vi "MeasurementSpin2String.vi"(1 "Seconds after Spin Stop":dbl[unit]=1.0, 2 "Seconds to Spin Start":dbl[unit]=1.0, 3 "Program Spin Coater":T1(array[cluster])) -> (0 "concatenated string":string)   [LabVIEW 2020]
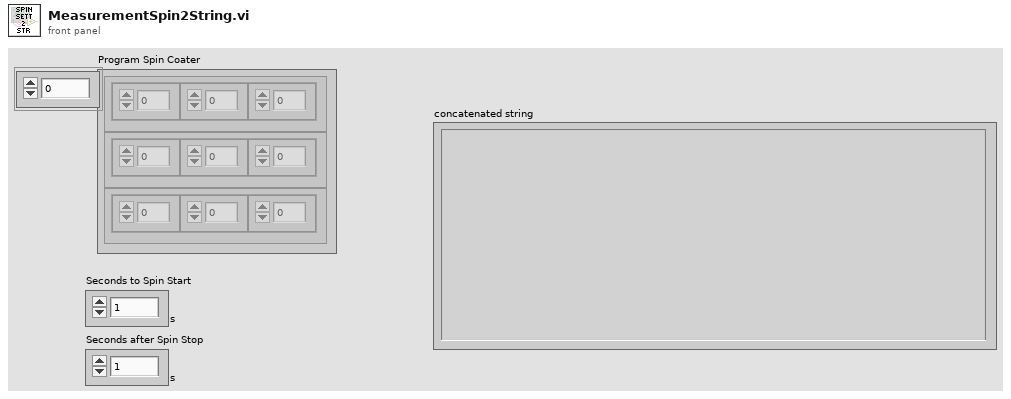
[diagram p1: front panel]
types:
  T1 = cluster{"Speed (rpm)":dbl, "Time (s)":dbl, "Acc (rpm/s)":dbl}[]
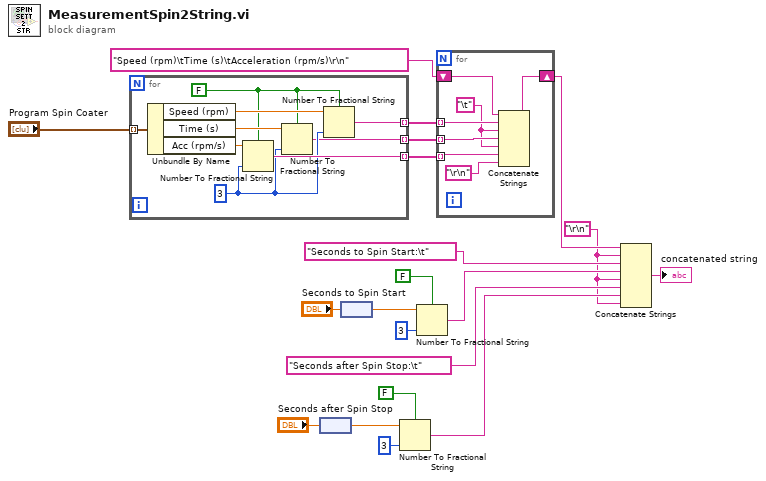
[diagram p0: block diagram]
diagram:
  w2 = "\r\n"
  n1 = for {
    tunnel: [w29] -> w19 mode=indexing
    tunnel: [w28] -> w17 mode=indexing
    tunnel: "Program Spin Coater" -> [w26] mode=indexing
    tunnel: [w23] -> w18 mode=indexing
    w27 = i16 3 ("precision (6)")
    w21 = FALSE ("use system decimal point (T)")
    n2 = Unbundle By Name(w26) -> ("Speed (rpm)"=w25:dbl, "Time (s)"=w24:dbl, "Acc (rpm/s)"=w22:dbl)
    n3 = Number To Fractional String(use system decimal point (T)=w21, number=w22, precision (6)=w27) -> (F-format string=w28:string)  [unwired: 1 in]
    n4 = Number To Fractional String(use system decimal point (T)=w21, number=w24, precision (6)=w27) -> (F-format string=w23:string)  [unwired: 1 in]
    n5 = Number To Fractional String(use system decimal point (T)=w21, number=w25, precision (6)=w27) -> (F-format string=w29:string)  [unwired: 1 in]
  }
  n6 = node("Seconds after Spin Stop") -> (w14:dbl)
  n7 = node("Seconds to Spin Start") -> (w12:dbl)
  n8 = Number To Fractional String(use system decimal point (T)=FALSE, number=w14, precision (6)=i16 3) -> (F-format string=w3:string)  [unwired: 1 in]
  n9 = Number To Fractional String(use system decimal point (T)=FALSE, number=w12, precision (6)=i16 3) -> (F-format string=w5:string)  [unwired: 1 in]
  n10 = for {
    tunnel: w19 -> [w36] mode=indexing
    tunnel: w18 -> [w35] mode=indexing
    tunnel: w17 -> [w33] mode=indexing
    shift-right: [w31] -> w7
    shift-left: "Speed (rpm)\tTime (s)\tAcceleration (rpm/s)\r\n" -> [w32]
    w34 = "\t"
    n11 = Concatenate Strings(w32, w36, w34, w35, w34, w33, "\r\n") -> (w31:string)
  }
  n12 = Concatenate Strings(w7, w2, "Seconds to Spin Start:\t", w5, w2, "Seconds after Spin Stop:\t", w3, w2) -> (→"concatenated string":string)
